vi "test_obj.vi"() -> ()   [LabVIEW 2021]
uses:
  model/refDll.dll
panel:
  in  "val 2":u64=6
  out "result":u64
  in  "val":u64=3
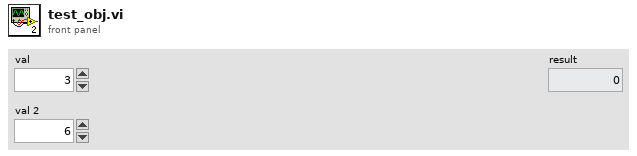
[diagram p1: front panel]
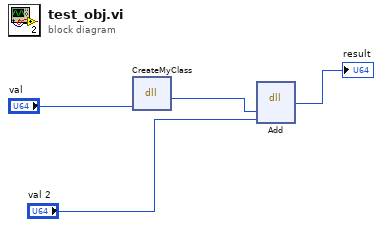
[diagram p0: block diagram]
diagram:
  n1 = dll-call lib="D:/labviewTestTCVdll/TransformCV-LabVIEW/Test/model/refDll.dll" fn="CreateMyClass"("val"="val") -> ("obj"=w3:u64)  [unwired: 4 in, 2 out]
  n2 = dll-call lib="D:/labviewTestTCVdll/TransformCV-LabVIEW/Test/model/refDll.dll" fn="Add"("ref"=w3, "val"="val 2") -> ("result"=→"result":u64)  [unwired: 5 in, 2 out]
